vi "Format Commands to Tree.vi"(8 "Paths":path[](array[path])=[path "C:/Users/gam.AMER/Documents/2468 code/trunk/FRC/2019/Software/2019 robot/Drive/Commands/Drive for Time.vi", path "C:/Users/gam.AMER/Documents/2468 code/trunk/FRC/2019/Software/2019 robot/Drive/Commands/Drive Immediate.vi", path "C:/Users/gam.AMER/Documents/2468 code/trunk/FRC/2019/Software/2019 robot/Drive/Commands/J-Turn.vi", path "C:/Users/gam.AMER/Documents/2468 code/trunk/FRC/2019/Software/2019 robot/Drive/Commands/Play Path.vi", path "C:/Users/gam.AMER/Documents/2468 code/trunk/FRC/2019/Software/2019 robot/Drive/Commands/Read Drive Operation.vi", path "C:/Users/gam.AMER/Documents/2468 code/trunk/FRC/2019/Software/2019 robot/Drive/Commands/Reserve Drive.vi", path "C:/Users/gam.AMER/Documents/2468 code/trunk/FRC/2019/Software/2019 robot/Drive/Commands/Stop Driving.vi", path "C:/Users/gam.AMER/Documents/2468 code/trunk/FRC/2019/Software/2019 robot/Drive/Commands/Template for Drive Immediate with Deadband.vit", path "C:/Users/gam.AMER/Documents/2468 code/trunk/FRC/2019/Software/2019 robot/Drive/Commands/Template for Drive Immediate.vit", path "C:/Users/gam.AMER/Documents/2468 code/trunk/FRC/2019/Software/2019 robot/Drive/Commands/Template for Drive with Duration.vit", path "C:/Users/gam.AMER/Documents/2468 code/trunk/FRC/2019/Software/2019 robot/Climb/Commands/climb.vi", path "C:/Users/gam.AMER/Documents/2468 code/trunk/FRC/2019/Software/2019 robot/Climb/Commands/Read Climb Operation.vi", path "C:/Users/gam.AMER/Documents/2468 code/trunk/FRC/2019/Software/2019 robot/Climb/Commands/Reserve Climb.vi", path "C:/Users/gam.AMER/Documents/2468 code/trunk/FRC/2019/Software/2019 robot/Climb/Commands/Template for Climb Immediate with Deadband.vit", path "C:/Users/gam.AMER/Documents/2468 code/trunk/FRC/2019/Software/2019 robot/Climb/Commands/Template for Climb Immediate.vit", path "C:/Users/gam.AMER/Documents/2468 code/trunk/FRC/2019/Software/2019 robot/Climb/Commands/Template for Climb with Duration.vit", path "C:/Users/gam.AMER/Documents/2468 code/trunk/FRC/2019/Software/2019 robot/Elevator/Commands/Elevator Immediate.vi", path "C:/Users/gam.AMER/Documents/2468 code/trunk/FRC/2019/Software/2019 robot/Elevator/Commands/Read Elevator Operation.vi", path "C:/Users/gam.AMER/Documents/2468 code/trunk/FRC/2019/Software/2019 robot/Elevator/Commands/Reserve Elevator.vi", path "C:/Users/gam.AMER/Documents/2468 code/trunk/FRC/2019/Software/2019 robot/Elevator/Commands/Template for Elevator Immediate with Deadband.vit", path "C:/Users/gam.AMER/Documents/2468 code/trunk/FRC/2019/Software/2019 robot/Elevator/Commands/Template for Elevator Immediate.vit", path "C:/Users/gam.AMER/Documents/2468 code/trunk/FRC/2019/Software/2019 robot/Elevator/Commands/Template for Elevator with Duration.vit", path "C:/Users/gam.AMER/Documents/2468 code/trunk/FRC/2019/Software/2019 robot/Floating Intake/Commands/Duration Intake.vi", path "C:/Users/gam.AMER/Documents/2468 code/trunk/FRC/2019/Software/2019 robot/Floating Intake/Commands/Floating Intake Immediate.vi", path "C:/Users/gam.AMER/Documents/2468 code/trunk/FRC/2019/Software/2019 robot/Floating Intake/Commands/Floating Intake Read.vi", path "C:/Users/gam.AMER/Documents/2468 code/trunk/FRC/2019/Software/2019 robot/Floating Intake/Commands/Read Floating Intake Operation.vi", path "C:/Users/gam.AMER/Documents/2468 code/trunk/FRC/2019/Software/2019 robot/Floating Intake/Commands/Reserve Floating Intake.vi", path "C:/Users/gam.AMER/Documents/2468 code/trunk/FRC/2019/Software/2019 robot/Floating Intake/Commands/Template for Floating Intake Immediate with Deadband.vit", path "C:/Users/gam.AMER/Documents/2468 code/trunk/FRC/2019/Software/2019 robot/Floating Intake/Commands/Template for Floating Intake Immediate.vit", path "C:/Users/gam.AMER/Documents/2468 code/trunk/FRC/2019/Software/2019 robot/Floating Intake/Commands/Template for Floating Intake with Duration.vit", path "C:/Users/gam.AMER/Documents/2468 code/trunk/FRC/2019/Software/2019 robot/Carriage Intake/Commands/Carriage Intake Immediate with Deadband.vi", path "C:/Users/gam.AMER/Documents/2468 code/trunk/FRC/2019/Software/2019 robot/Carriage Intake/Commands/Carriage Intake Immediate.vi", path "C:/Users/gam.AMER/Documents/2468 code/trunk/FRC/2019/Software/2019 robot/Carriage Intake/Commands/Read Carriage Intake Operation.vi", path "C:/Users/gam.AMER/Documents/2468 code/trunk/FRC/2019/Software/2019 robot/Carriage Intake/Commands/Reserve Carriage Intake.vi", path "C:/Users/gam.AMER/Documents/2468 code/trunk/FRC/2019/Software/2019 robot/Carriage Intake/Commands/Template for Carriage Intake Immediate with Deadband.vit", path "C:/Users/gam.AMER/Documents/2468 code/trunk/FRC/2019/Software/2019 robot/Carriage Intake/Commands/Template for Carriage Intake Immediate.vit", path "C:/Users/gam.AMER/Documents/2468 code/trunk/FRC/2019/Software/2019 robot/Carriage Intake/Commands/Template for Carriage Intake with Duration.vit", path "C:/Users/gam.AMER/Documents/2468 code/trunk/FRC/2019/Software/2019 robot/LattePanda/Commands/Is Connected.vi", path "C:/Users/gam.AMER/Documents/2468 code/trunk/FRC/2019/Software/2019 robot/LattePanda/Commands/Power On.vi", path "C:/Users/gam.AMER/Documents/2468 code/trunk/FRC/2019/Software/2019 robot/LattePanda/Commands/Read LattePanda Operation.vi", path "C:/Users/gam.AMER/Documents/2468 code/trunk/FRC/2019/Software/2019 robot/LattePanda/Commands/Reserve LattePanda.vi", path "C:/Users/gam.AMER/Documents/2468 code/trunk/FRC/2019/Software/2019 robot/LattePanda/Commands/Shut Down.vi", path "C:/Users/gam.AMER/Documents/2468 code/trunk/FRC/2019/Software/2019 robot/LattePanda/Commands/Template for LattePanda Immediate with Deadband.vit", path "C:/Users/gam.AMER/Documents/2468 code/trunk/FRC/2019/Software/2019 robot/LattePanda/Commands/Template for LattePanda Immediate.vit", path "C:/Users/gam.AMER/Documents/2468 code/trunk/FRC/2019/Software/2019 robot/LattePanda/Commands/Template for LattePanda with Duration.vit"], 9 "Command Info":T4(array[cluster]), 11 "Tree Refnum":refnum<vi>) -> (2 "2D Picture":picture, 3 "Filtered Command Info Out":T1)   [LabVIEW 2023]
uses:
  <vilib>/picture/picture.llb/imagedata.ctl
  Types/Command Editor Info.ctl
  Types/Single Cmd Info.ctl
  <vilib>/Utility/Data Type/NI_Data Type.lvlib
panel:
  in  "Tree":string(tree)
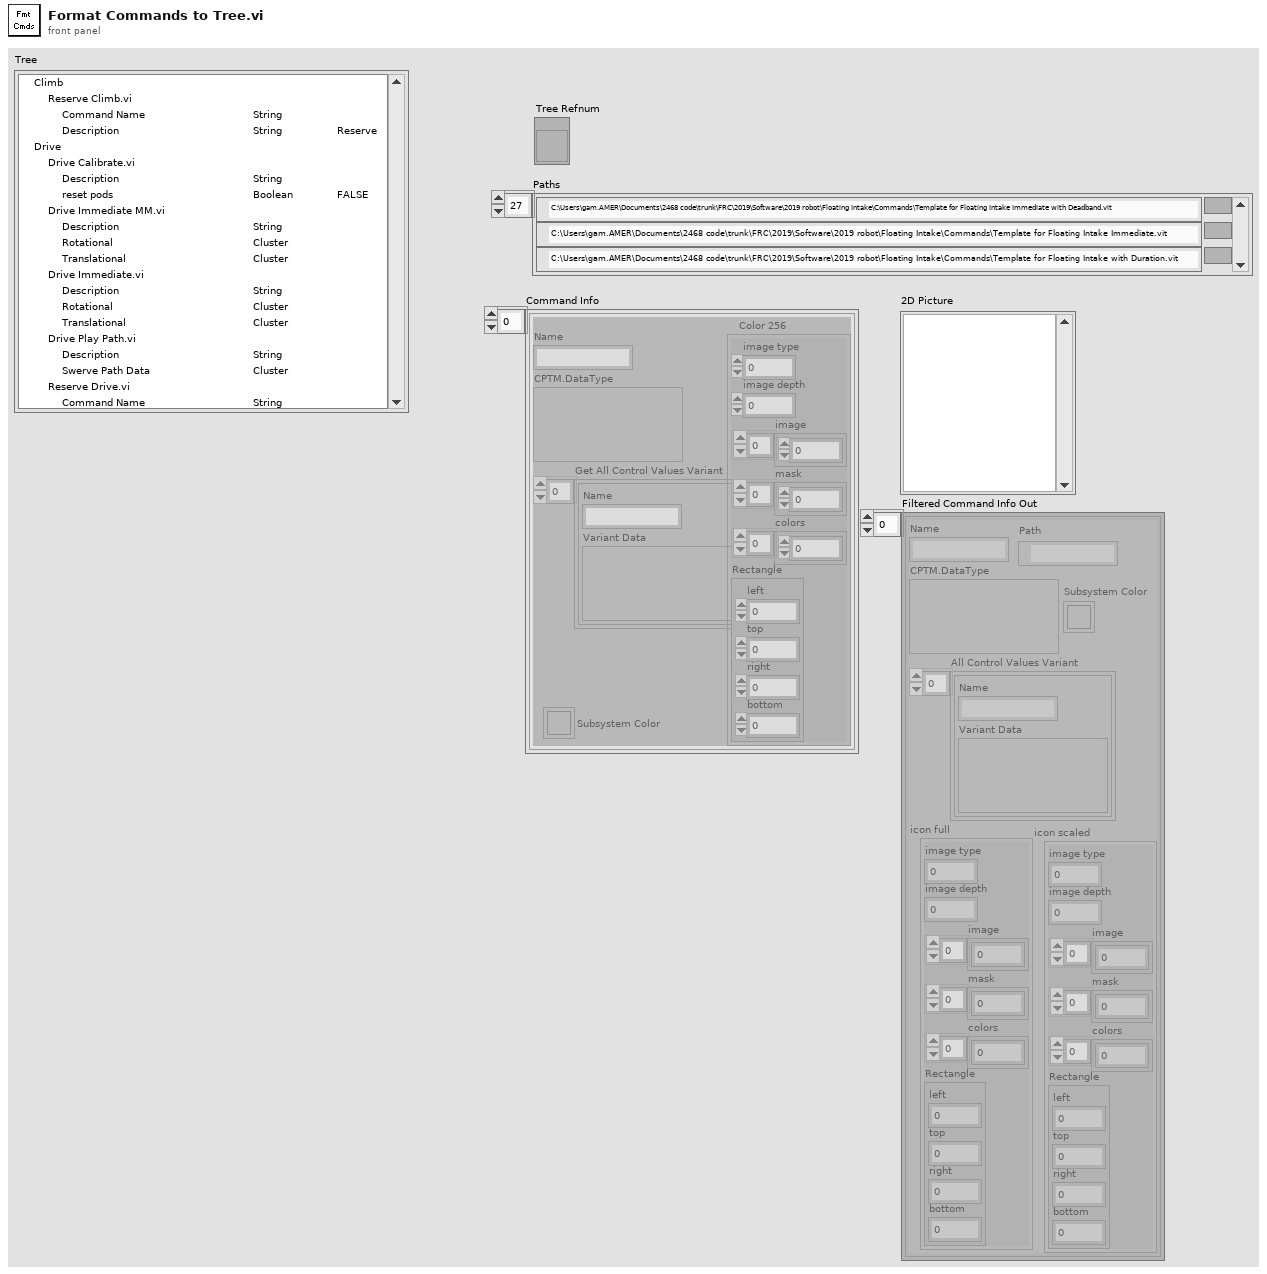
[diagram p1: front panel]
types:
  T1 = typedef "Command Editor Info.ctl" = T2[]
  T2 = typedef "Single Cmd Info.ctl" = cluster{"Name":string, "CPTM.DataType":variant, "All Control Values Variant":cluster{"Name":string, "Variant Data":variant}[], "icon full":T3, "icon scaled":T3, "Path":path, "Subsystem Color":u32}
  T3 = typedef "imagedata.ctl" = cluster{"image type":i32, "image depth":i32, "image":u8[], "mask":u8[], "colors":u32[], "Rectangle":cluster{"left":i16, "top":i16, "right":i16, "bottom":i16}}
  T4 = cluster{"Name":string, "CPTM.DataType":variant, "Get All Control Values Variant":cluster{"Name":string, "Variant Data":variant}[], "Color 256":T3, "Subsystem Color":u32}[]
  T5 = cluster{"Left Cell String":string, "Child Text":string[], "Child Tag":string, "Item Indent":i32, "Child Only?":bool, "Glyph Index":i32}
  T6 = cluster{"Left Cell String":string, "Child Text":string[], "Child Tag":string, "Item Indent":i32, "Child Only?":bool, "Glyph Index":i32}[]
  T7 = cluster{"Name":string, "CPTM.DataType":variant, "Get All Control Values Variant":cluster{"Name":string, "Variant Data":variant}[], "Color 256":T3, "Color 256":T3, "Path":path, "Subsystem Color":u32}
  T8 = typedef "NI_Data Type.lvlib/Data Type.ctl" = enum8{"Invalid Type", "Void", "I8", "I16", "I32", "I64", "U8", "U16", "U32", "U64", "Single Float", "Double Float", "Extended Float", "Single Complex", "Double Complex", "Extended Complex", "Enum U8", "Enum U16", "Enum U32", "Enum U64", "Single Float With Unit", "Double Float With Unit", "Extended Float With Unit", "Single Complex with Unit", "Double Complex with Unit", "Extended Complex with Unit", "Boolean", "String", "Path", "Picture", "Tag", "Array", "Cluster", "Variant", "LV Variant", "Waveform", "Timestamp", "Digital Waveform", "Digital Data", "ExpressData", "Refnum", "External Data", "VI", "Poly VI", "LabVIEW Class Instance", "Fixed Point", "Set Collection", "Map Collection"}
  T9 = typedef "NI_Data Type.lvlib/Type Definition Info.ctl" = cluster{"Name":string, "Timestamp":u32}
  T10 = cluster{"left":i16, "top":i16, "right":i16, "bottom":i16}
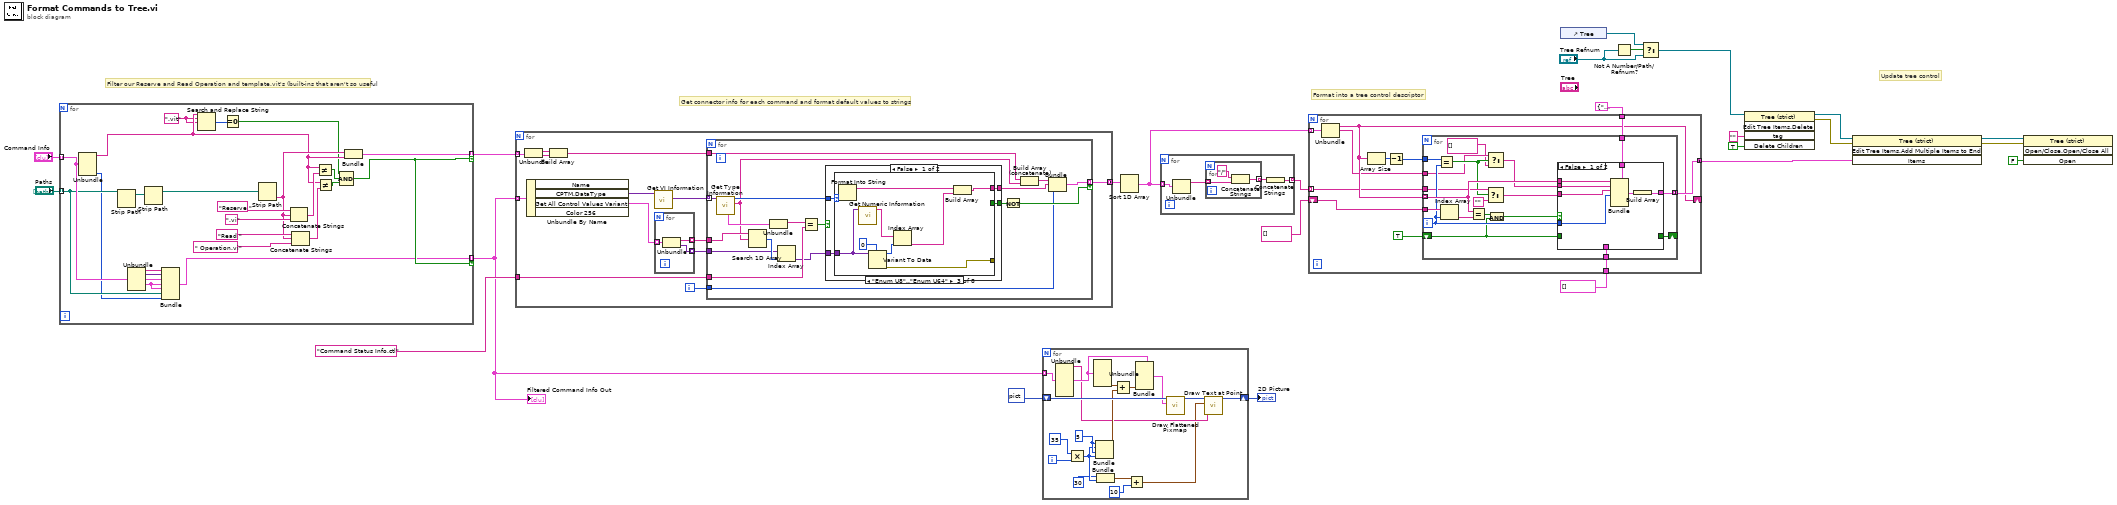
[diagram p0: block diagram]
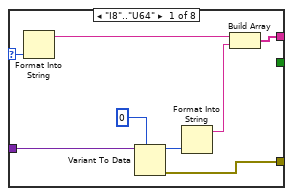
[diagram p2: hidden frame]
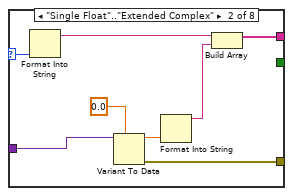
[diagram p3: hidden frame]
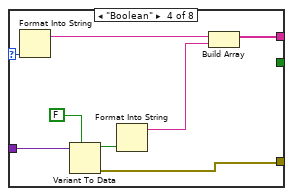
[diagram p4: hidden frame]
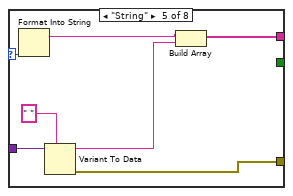
[diagram p5: hidden frame]
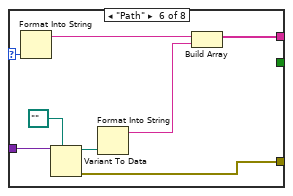
[diagram p6: hidden frame]
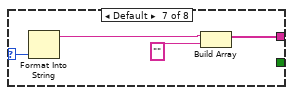
[diagram p7: hidden frame]
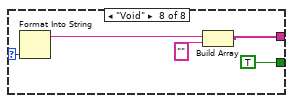
[diagram p8: hidden frame]
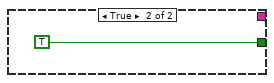
[diagram p9: hidden frame]
diagram:
  # "Update tree control"
  # "Get connector info for each command and format default values to strings"
  # "Filter our Reserve and Read Operation and template.vit's (built-ins that aren't so useful"
  # "Format into a tree control descriptor"
  n1 = for {
    tunnel: "Command Info" -> [w37] mode=indexing
    tunnel: "Paths" -> [w36] mode=indexing
    tunnel: [w48] -> w2 mode=indexing if=w47
    tunnel: [w38] -> w1 mode=indexing if=w47
    w29 = ".vit" ("search string")
    n2 = Unbundle(w37) -> ("Name"=w30:string, "Subsystem Color"=w35:u32)  [unwired: 3 out]
    n3 = Strip Path(path=w36) -> (stripped path=w50:path)  [unwired: 1 out]
    n4 = Unbundle(w37) -> ("Name"=w39:string, "CPTM.DataType"=w40:variant, "Get All Control Values Variant"=w41:cluster{"Name":string, "Variant Data":variant}[], "Color 256"=w42:T3)  [unwired: 1 out]
    n5 = Strip Path(path=w50) -> (stripped path=w49:path)  [unwired: 1 out]
    n6 = Bundle("Name"=w39, "CPTM.DataType"=w40, "Get All Control Values Variant"=w41, "Color 256"=w42, "Color 256"=w42, "Path"=w36, "Subsystem Color"=w35) -> (w38:T7)  [unwired: 1 in]
    n7 = Search and Replace String(input string=w30, search string=w29, replace string=w29) -> (number of replacements=w28:i32)  [unwired: 5 in, 3 out]
    n8 = Equal To 0?(x=w28) -> (x = 0?=w27:bool)
    n9 = Strip Path(path=w49) -> (name=w33:string)  [unwired: 1 out]
    n10 = Concatenate Strings("Reserve ", w33, ".vi") -> (w34:string)
    n11 = Concatenate Strings("Read ", w33, " Operation.vi") -> (w32:string)
    n12 = Not Equal?(x=w30, y=w34) -> (x != y?=w26:bool)
    n13 = Not Equal?(x=w30, y=w32) -> (x != y?=w31:bool)
    n14 = Compound Arithmetic op=AND(w27, w26, w31) -> (w47:bool)
    n15 = Bundle("name"=w33, "Name"=w30) -> (w48:cluster{"name":string, "Name":string})  [unwired: 1 in]
  }
  "Filtered Command Info Out" <- w1
  n16 = for {
    tunnel: w2 -> [w63] mode=indexing
    tunnel: [w56] -> w22 mode=concatenating
    tunnel: w1 -> [w60] mode=indexing
    tunnel: "Command Status Info.ctl" ("Name") -> [w55]
    i -> [w51]
    n17 = Unbundle(w63) -> ("name"=w62:string, "Name"=w61:string)
    n18 = Unbundle By Name(w60) -> ("CPTM.DataType"=w59:variant, "Get All Control Values Variant"=w54:cluster{"Name":string, "Variant Data":variant}[])  [unwired: 2 out]
    n19 = Build Array(w62, w61) -> (w58:string[])
    n20 = call <vilib>:"Get VI Information.vi"("variant"=w59) -> ("VI terminal types"=w57:variant[])  [unwired: 7 in, 3 out]
    n21 = for {
      tunnel: w54 -> [w66] mode=indexing
      tunnel: [w65] -> w53 mode=indexing
      tunnel: [w64] -> w52 mode=indexing
      n22 = Unbundle(w66) -> ("Name"=w65:string, "Variant Data"=w64:variant)
    }
    n23 = for {
      tunnel: w58 -> [w82]
      tunnel: w57 -> [w84] mode=indexing
      tunnel: [w80] -> w56 mode=indexing if=w74
      tunnel: w55 -> [w78]
      tunnel: w53 -> [w72]
      tunnel: w52 -> [w69]
      tunnel: w51 -> [w67]
      n24 = call <vilib>:"Get Type Information.vi"("variant"=w84) -> ("name"=w71:string, "type"=w83:T8, "type definition info"=w79:T9)  [unwired: 6 in, 2 out]
      n25 = Search 1D Array(1D array=w72, element=w71) -> (index of element=w70:i32)  [unwired: 1 in]
      n26 = Unbundle(w79) -> ("Name"=w77:string)  [unwired: 1 out]
      n27 = Index Array(array=w69, index=w70) -> (element=w68:variant)
      n28 = Equal?(x=w77, y=w78) -> (x = y?=w76:bool)
      n29 = case shown="False" w76 {
        tunnel: w83 -> [w88 _]
        tunnel: [w87 _] -> w73
        tunnel: [w86 TRUE] -> w75
        tunnel: w68 -> [w85 _]
        frame False {
          n30 = case shown="\"Enum U8\"..\"Enum U64\"" w88 {
            selector: w88 -> [w96 w104 w113 w121 w128 w136 w140 w145]
            tunnel: [w91 w98 w110 w116 w125 w131 w138 w142] -> w87
            tunnel: [_ _ _ _ _ _ _ TRUE] -> w86
            tunnel: w85 -> [w90 w101 w108 w118 w127 w133 _ _]
            tunnel: [w89 w97 w109 w114 w122 w129 _ _] -> _
            frame "I8".."U64" {
              n31 = Format Into String(w96) -> (resulting string=w92:string)  [unwired: 3 in, 1 out]
              n32 = Variant To Data(type=i64 0, Variant=w90) -> (data=w94:i64, error out=w89:errorcluster)  [unwired: 1 in]
              n33 = Format Into String(w94) -> (resulting string=w93:string)  [unwired: 3 in, 1 out]
              n34 = Build Array(w92, w93) -> (w91:string[])
            }
            frame "Single Float".."Extended Complex" {
              n35 = Format Into String(w104) -> (resulting string=w100:string)  [unwired: 3 in, 1 out]
              n36 = Variant To Data(type=0.0, Variant=w101) -> (data=w102:dbl, error out=w97:errorcluster)  [unwired: 1 in]
              n37 = Format Into String(w102) -> (resulting string=w99:string)  [unwired: 3 in, 1 out]
              n38 = Build Array(w100, w99) -> (w98:string[])
            }
            frame "Enum U8".."Enum U64" {
              n39 = Format Into String(w113) -> (resulting string=w111:string)  [unwired: 3 in, 1 out]
              n40 = call <vilib>:"Get Numeric Information.vi"("variant"=w108) -> ("enum names"=w107:string[])  [unwired: 7 in, 3 out]
              n41 = Variant To Data(type=i64 0, Variant=w108) -> (data=w106:i64, error out=w109:errorcluster)  [unwired: 1 in]
              n42 = Index Array(array=w107, index=w106) -> (element=w105:string)
              n43 = Build Array(w111, w105) -> (w110:string[])
            }
            frame "Boolean" {
              n44 = Format Into String(w121) -> (resulting string=w117:string)  [unwired: 3 in, 1 out]
              n45 = Variant To Data(type=FALSE, Variant=w118) -> (data=w119:bool, error out=w114:errorcluster)  [unwired: 1 in]
              n46 = Format Into String(w119) -> (resulting string=w115:string)  [unwired: 3 in, 1 out]
              n47 = Build Array(w117, w115) -> (w116:string[])
            }
            frame "String" {
              n48 = Format Into String(w128) -> (resulting string=w126:string)  [unwired: 3 in, 1 out]
              n49 = Variant To Data(type=" ", Variant=w127) -> (data=w124:string, error out=w122:errorcluster)  [unwired: 1 in]
              n50 = Build Array(w126, w124) -> (w125:string[])
            }
            frame "Path" {
              n51 = Format Into String(w136) -> (resulting string=w132:string)  [unwired: 3 in, 1 out]
              n52 = Variant To Data(type=path "", Variant=w133) -> (data=w134:path, error out=w129:errorcluster)  [unwired: 1 in]
              n53 = Format Into String(w134) -> (resulting string=w130:string)  [unwired: 3 in, 1 out]
              n54 = Build Array(w132, w130) -> (w131:string[])
            }
            frame Default {
              n55 = Format Into String(w140) -> (resulting string=w139:string)  [unwired: 3 in, 1 out]
              n56 = Build Array(w139, "") -> (w138:string[])
            }
            frame "Void" {
              n57 = Format Into String(w145) -> (resulting string=w143:string)  [unwired: 3 in, 1 out]
              n58 = Build Array(w143, "") -> (w142:string[])
            }
          }
        }
        frame True {
        }
      }
      n59 = Not(x=w75) -> (.not. x?=w74:bool)
      n60 = Build Array (concatenate)(w82, w71) -> (w81:string[])
      n61 = Bundle(w81, w73, w67) -> (w80:cluster{string[], string[], i32})  [unwired: 1 in]
    }
  }
  n62 = for {
    tunnel: w1 -> [w163] mode=indexing
    shift-right: [w154] -> w3
    shift-left: picture data[5B] ("2D Picture") -> [w164]
    i -> [w159]
    w158 = 5
    n63 = Unbundle(w163) -> ("Name"=w150:string, "Color 256"=w162:T3)  [unwired: 5 out]
    n64 = Multiply(x=35, y=w159) -> (x*y=w152:i32)
    n65 = Unbundle(w162) -> ("Rectangle"=w160:T10)  [unwired: 5 out]
    n66 = Bundle(w158, w152, w158, w152) -> (w157:cluster{i32, i32, i32, i32})  [unwired: 1 in]
    n67 = Bundle(30, w152) -> (w149:cluster{i32, i32})  [unwired: 1 in]
    n68 = Add(x=w160, y=w157) -> (x+y=w156:cluster{i32, i32, i32, i32})
    n69 = Add(x=w149, y=10) -> (x+y=w148:cluster{i32, i32})
    n70 = Bundle(cluster=w162, "Rectangle"=w156) -> (w161:T3)  [unwired: 5 in]
    n71 = call <vilib>:"Draw Flattened Pixmap.vi"("image data"=w161, "picture"=w164) -> ("new picture"=w155:picture)  [unwired: 7 in]
    n72 = call <vilib>:"Draw Text at Point.vi"("text"=w150, "origin"=w148, "picture"=w155) -> ("new picture"=w154:picture)  [unwired: 7 in, 1 out]
  }
  "2D Picture" <- w3
  n73 = Sort 1D Array(array=w22) -> (sorted array=w23:cluster{string[], string[], i32}[])
  n74 = for {
    tunnel: w23 -> [w168] mode=indexing
    tunnel: [w165] -> w24 mode=indexing
    n75 = Unbundle(w168) -> (w167:string[])  [unwired: 2 out]
    n76 = for {
      tunnel: w167 -> [w170] mode=indexing
      tunnel: [w169] -> w166 mode=indexing
      n77 = Concatenate Strings("/", w170) -> (w169:string)
    }
    n78 = Concatenate Strings(w166) -> (w165:string)
  }
  n79 = for {
    tunnel: [w178] -> w25 mode=concatenating
    tunnel: T5 {"Left Cell String"="", "Child Text"=[], "Child Tag"="", "Item Indent"=0, "Child Only?"=FALSE, "Glyph Index"=0} ("Item") -> [w179]
    shift-right: [w175] -> _
    shift-left: string[] [] ("Child Text") -> [w181]
    tunnel: w23 -> [w182] mode=indexing
    tunnel: T6 [] -> [w180]
    tunnel: w24 -> [w174] mode=indexing
    n80 = Unbundle(w182) -> (w175:string[], w172:string[])  [unwired: 1 out]
    n81 = Array Size(array=w175) -> (size(s)=w177:i32)
    n82 = Decrement(x=w177) -> (x-1=w176:i32)
    n83 = for {
      tunnel: w181 -> [w201]
      tunnel: w175 -> [w196] mode=indexing
      tunnel: w180 -> [w199]
      tunnel: [w198] -> w178 mode=concatenating
      tunnel: w179 -> [w197]
      tunnel: w176 -> [w194]
      tunnel: w172 -> [w184]
      tunnel: w174 -> [w192]
      shift-right: [w188] -> _
      shift-left: TRUE -> [w187]
      i -> [w195]
      n84 = Equal?(x=w194, y=w195) -> (x = y?=w185:bool)
      n85 = Index Array(array=w201, index=w195) -> (element=w200:string)
      n86 = Equal?(x=w196, y=w200) -> (x = y?=w190:bool)
      n87 = Select(t=w192, s=w185, f="") -> (s? t:f=w193:string)
      n88 = Select(t=w184, s=w185, f=string[] [] ("appended array")) -> (s? t:f=w186:string[])
      n89 = And(x=w190, y=w187) -> (x .and. y?=w189:bool)
      n90 = case shown="False" w189 {
        tunnel: [w206 w210] -> w198
        tunnel: w199 -> [_ w210]
        tunnel: w197 -> [w208 _]
        tunnel: w196 -> [w205 _]
        tunnel: w195 -> [w204 _]
        tunnel: w186 -> [w203 _]
        tunnel: w193 -> [w202 _]
        tunnel: [_ w209] -> w188
        tunnel: w187 -> [_ w209]
        frame False {
          n91 = Bundle(cluster=w208, "Left Cell String"=w205, "Child Text"=w203, "Child Tag"=w202, "Item Indent"=w204) -> (w207:T5)  [unwired: 2 in]
          n92 = Build Array(w207) -> (w206:T6)
        }
        frame True {
        }
      }
    }
  }
  n93 = control-ref of="Tree"() -> (w6:refnum<vi>)
  n94 = Not A Number/Path/Refnum?(number/path/refnum="Tree Refnum") -> (NaN/Path/Refnum?=w10:bool)
  n95 = Select(t=w6, s=w10, f="Tree Refnum") -> (s? t:f=w9:refnum<vi>)
  n96 = invoke on="Invoke Node" class="Tree (strict)" method="Edit Tree Items.Delete"(reference=w9, "tag"="" ("Tag"), "Delete Children"=TRUE ("Delete Children?")) -> (reference out=w8:refnum<vi>, error out=w15:errorcluster)  [unwired: 2 in, 3 out]
  n97 = invoke on="Invoke Node" class="Tree (strict)" method="Edit Tree Items.Add Multiple Items to End"(reference=w8, error in=w15, "Items"=w25) -> (reference out=w7:refnum<vi>, error out=w12:errorcluster)  [unwired: 1 in, 2 out]
  n98 = invoke on="Invoke Node" class="Tree (strict)" method="Open/Close.Open/Close All"(reference=w7, error in=w12, "Open"=FALSE ("Open?")) -> ()  [unwired: 1 in, 4 out]
